vi "Create (String Array).vi"(6 "timestamp in":timestamp, 8 "error in (no error)":errorcluster, 10 "value in":string[](array[string])) -> (0 "error out":errorcluster, 2 "value out":string[](array[string]), 3 "NT Scalar out":refnum<class "NT Scalar.lvclass">, 4 "timestamp out":timestamp)   [LabVIEW 2020, in "PV Access.lvlib" / "PV Data.lvlib" / "NT Scalar.lvclass"]
uses:
  NT Scalar.lvclass
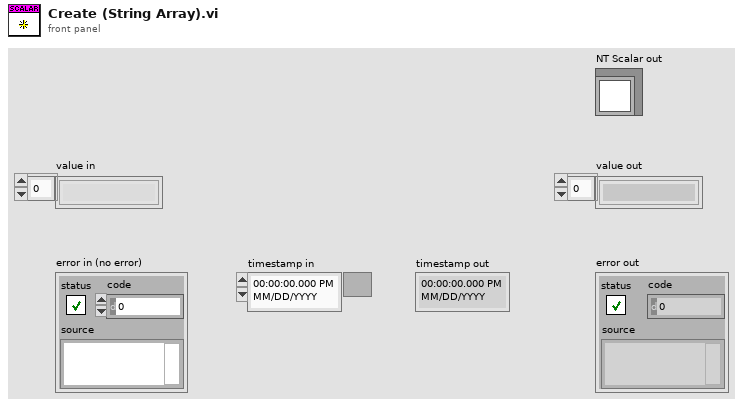
[diagram p1: front panel]
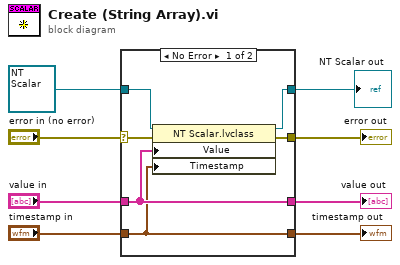
[diagram p0: block diagram]
diagram:
  n1 = case shown="No Error" "error in (no error)" {
    selector: "error in (no error)" -> [w12 w18]
    tunnel: [w11 w18] -> w7
    tunnel: [w13 w17] -> w5
    tunnel: refnum<class "NT Scalar.lvclass"> refnum ("NT Scalar in") -> [w14 w17]
    tunnel: "value in" -> [w10 w16]
    tunnel: "timestamp in" -> [w9 w15]
    tunnel: [w10 w16] -> w3
    tunnel: [w9 w15] -> w2
    frame No Error {
      n2 = property class="NT Scalar.lvclass"(reference=w14, error in=w12, "Value"=w10, "Timestamp"=w9) -> (reference out=w13:refnum<class "NT Scalar.lvclass">, error out=w11:errorcluster)
    }
    frame Error {
    }
  }
  "error out" <- w7
  "NT Scalar out" <- w5
  "timestamp out" <- w2
  "value out" <- w3
